vi "rqcAlice Read DAC Level FIFO.vi"(7 "timeout (ms)":i32, 8 "error in":errorcluster, 9 "number of elements":u32, 10 "read all available":bool=TRUE, 11 "Alice FPGA Reference In":refnum<k20>) -> (0 "error out":errorcluster, 1 "TimeOut?":bool, 2 "Data":u8[](array[numeric]), 3 "Alice FPGA Reference Out":refnum<k20>)   [LabVIEW 2019]
uses:
  <vilib>/Utility/error.llb/Error Cluster From Error Code.vi
  <vilib>/rvi/errors/niLvFpgaAdjustHostInterfaceError.vi
  <vilib>/rvi/interface/nirviMethod/nirviMethod.xnode
  <vilib>/FPGAPlugInAG/Dynamic/niLvFpga_ReadFifo_Dynamic.vi
  <vilib>/rvi/errors/niLvFpgaMergeErrorWithErrorCode.vi
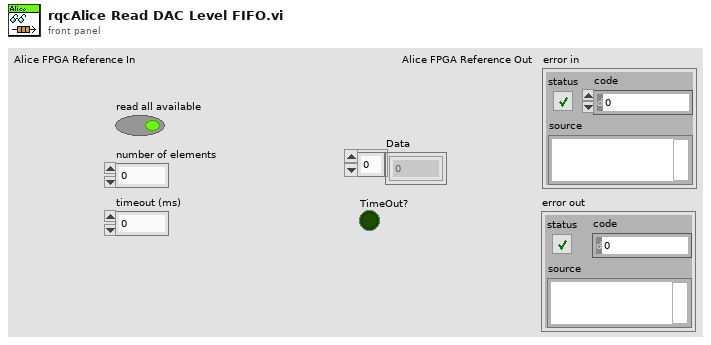
[diagram p1: front panel]
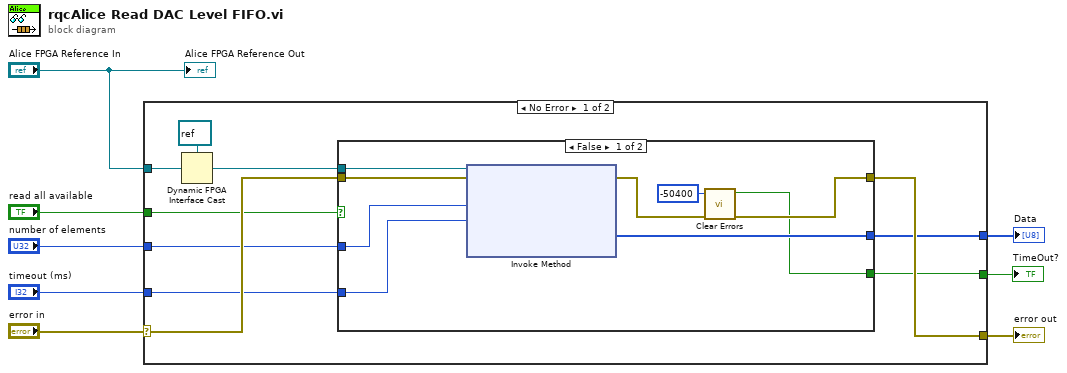
[diagram p0: block diagram]
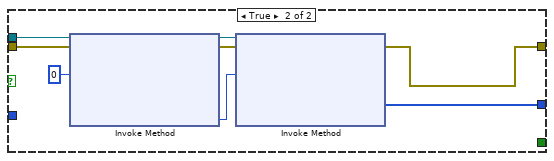
[diagram p2: hidden frame]
diagram:
  n1 = case shown="No Error" "error in" {
    selector: "error in" -> [w15 w36]
    tunnel: [w14 w36] -> w7
    tunnel: "Alice FPGA Reference In" -> [w18 _]
    tunnel: "number of elements" -> [w13 _]
    tunnel: "timeout (ms)" -> [w12 _]
    tunnel: "read all available" -> [w11 _]
    tunnel: [w10 _] -> w2
    tunnel: [w9 _] -> w1
    frame No Error {
      n2 = Dynamic FPGA Interface Cast(Session In=refnum<k20> refnum ("Type"), Type=w18) -> (Session Out=w16:refnum<k20>)
      n3 = case shown="False" w11 {
        tunnel: w13 -> [w25 _]
        tunnel: [w20 w28] -> w14
        tunnel: w16 -> [w27 w33]
        tunnel: w15 -> [w26 w32]
        tunnel: [w24 w29] -> w10
        tunnel: w12 -> [w23 _]
        tunnel: [w19 _] -> w9
        frame False {
          n4 = xnode "Invoke Method"("FPGA VI Reference In"=w27, "error in"=w26, "Number of Elements"=w25, "Timeout (ms)"=w23) -> ("error out"=w21:errorcluster, "Data"=w24:u8[])  [unwired: 2 out]
          n5 = call <vilib>:"Clear Errors.vi"("error in (no error)"=w21, "specific error code to clear (0: all)"=-50400) -> ("error out"=w20:errorcluster, "specific error cleared?"=w19:bool)  [unwired: 4 in]
        }
        frame True {
          n6 = xnode "Invoke Method"("FPGA VI Reference In"=w33, "error in"=w32, "Number of Elements"=u32 0) -> ("FPGA VI Reference Out"=w35:refnum<k20>, "error out"=w34:errorcluster, "Elements Remaining"=w31:u32)  [unwired: 1 in, 1 out]
          n7 = xnode "Invoke Method"("FPGA VI Reference In"=w35, "error in"=w34, "Number of Elements"=w31) -> ("error out"=w28:errorcluster, "Data"=w29:u8[])  [unwired: 1 in, 2 out]
        }
      }
    }
    frame Error {
    }
  }
  "error out" <- w7
  "Data" <- w2
  "TimeOut?" <- w1
  "Alice FPGA Reference Out" <- "Alice FPGA Reference In"
